vi "P3AT_Panel_Msg.vi"(8 "error in (no error)":errorcluster caption="错误输入（无错误）", 10 "值(信号)":T1={"max_vel"=0.49056603773584906, "max_rot"=0.5094339622641509, "Control_Mode"=enum."Joy"} {"max_rot" scale=0.0..1.0; "max_vel" scale=0.0..1.0}, 11 "RemoteP3AT输入":refnum<class "RemoteP3AT.lvclass">) -> (0 "error out":errorcluster caption="错误输出", 3 "RemoteP3AT输出":refnum<class "RemoteP3AT.lvclass">)   [LabVIEW 2014, in "RemoteP3AT.lvlib" / "RemoteP3AT.lvclass"]
uses:
  RemoteP3AT.lvclass
  ctl/P3AT_Panel.ctl
  RemoteP3AT.lvclass/RemoteP3AT.ctl
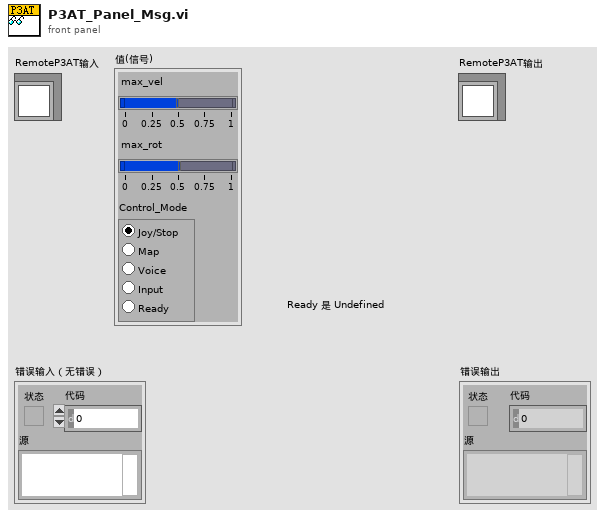
[diagram p1: front panel]
types:
  T1 = typedef "P3AT_Panel.ctl" = cluster{"max_vel":dbl, "max_rot":dbl, "Control_Mode":enum32{"Joy", "Map", "Voice", "Input", "Undefined"}}
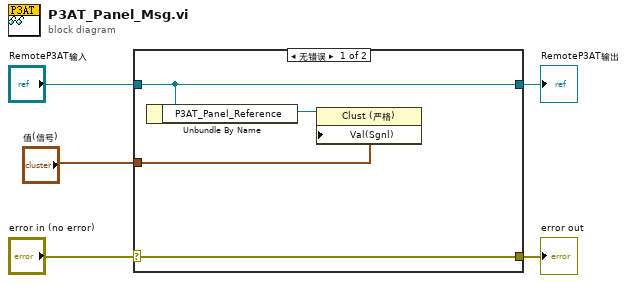
[diagram p0: block diagram]
diagram:
  n1 = case shown="无错误" "error in (no error)" {
    selector: "error in (no error)" -> [w9 w10]
    tunnel: [w9 w10] -> w4
    tunnel: [w8 w11] -> w2
    tunnel: "RemoteP3AT输入" -> [w8 w11]
    tunnel: "值(信号)" -> [w6 _]
    frame No Error {
      n2 = Unbundle By Name(w8) -> ("P3AT_Panel_Reference"=w7:refnum<vi>)
      n3 = property class="Clust (严格)"(reference=w7, "Val(Sgnl)"=w6) -> ()  [unwired: 1 in, 2 out]
    }
    frame Error {
    }
  }
  "error out" <- w4
  "RemoteP3AT输出" <- w2
